vi "Unregister Event.vi"(8 "Error In":errorcluster, 9 "Registrant Address":refnum<class "Message Enqueuer.lvclass">, 10 "Event":refnum<class "Event.lvclass">, 11 "Event Source In":refnum<class "Event Source.lvclass">) -> (0 "Error Out":errorcluster, 3 "Event Source Out":refnum<class "Event Source.lvclass">)   [LabVIEW 2016, in "Event Source.lvlib" / "Event Source.lvclass"]
doc: "This method unregisters a specific Actors Enqueuer from specific Event he is listening to, in this Event Source Actor."
uses:
  Event Source.lvclass
  <vilib>/ActorFramework/Message Enqueuer/Message Enqueuer.lvclass
  Event/Event.lvclass
  Event/Event.lvclass/Event.ctl
  Event Source.lvclass/Event Source.ctl
  <resource>/AFDebug/TDM Registry.vi
  <resource>/AFDebug/Localized Strings.vi
  <resource>/AFDebug/Actor Registry.vi
  <resource>/AFDebug/Get Clone Name.vi
  <resource>/AFDebug/AF Debug.lvlib
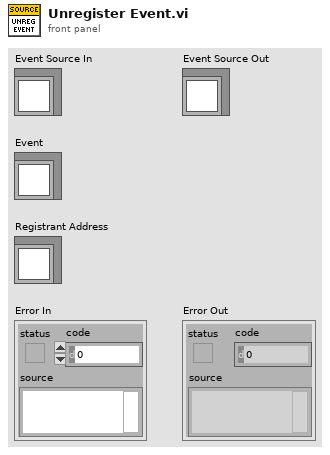
[diagram p1: front panel]
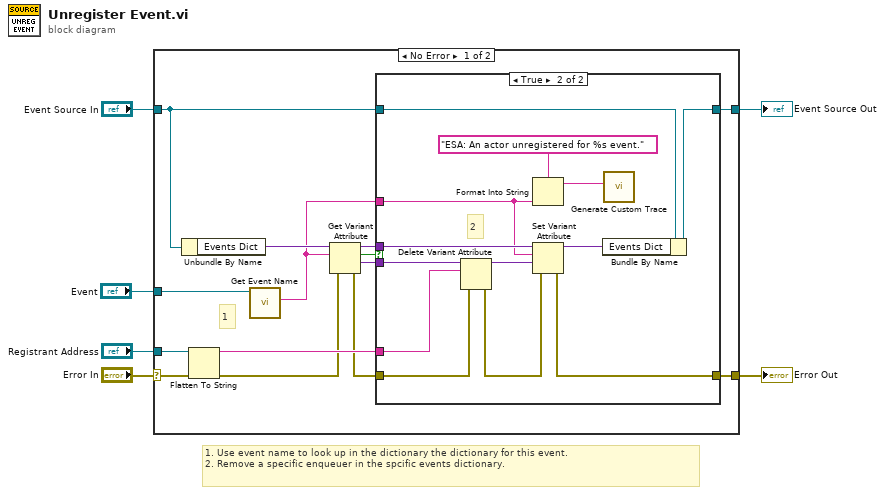
[diagram p0: block diagram]
diagram:
  # "1. Use event name to look up in the dictionary the dictionary for this event.\n2. Remove a specific enqueuer in the spcific events dictionary."
  n1 = case shown="No Error" "Error In" {
    selector: "Error In" -> [w17 w37]
    tunnel: "Registrant Address" -> [w20 _]
    tunnel: [w18 w37] -> w5
    tunnel: "Event" -> [w9 _]
    tunnel: "Event Source In" -> [w10 w36]
    tunnel: [w11 w36] -> w1
    frame No Error {
      # "1"
      n2 = Unbundle By Name(w10) -> ("Events Dict"=w16:variant)
      n3 = Flatten To String(anything=w20, error in (no error)=w17) -> (data string=w19:string, error out=w8:errorcluster)  [unwired: 2 in, 1 out]
      n4 = call "Get Event Name.vi"("Event In"=w9) -> ("Name"=w7:string)  [unwired: 9 in, 1 out]
      n5 = Get Variant Attribute(Variant=w16, name=w7, error in=w8) -> (duplicate Variant=w12:variant, found=w13:bool, value=w14:variant, error out=w15:errorcluster)  [unwired: 1 in]
      n6 = case shown="True" w13 {
        tunnel: w14 -> [_ w35]
        tunnel: w19 -> [_ w34]
        tunnel: w15 -> [w22 w33]
        tunnel: [w22 w29] -> w18
        tunnel: w12 -> [_ w32]
        tunnel: w7 -> [_ w23]
        tunnel: w10 -> [w21 w28]
        tunnel: [w21 w26] -> w11
        frame False {
        }
        frame True {
          # "2"
          n7 = Delete Variant Attribute(4:w33, 6:w34, 7:w35) -> (0:w30:errorcluster, 3:w31:variant)  [unwired: 1 out]
          n8 = Format Into String(format string="ESA: An actor unregistered for %s event." ("Custom Action"), w23) -> (resulting string=w24:string)  [unwired: 2 in, 1 out]
          n9 = Set Variant Attribute(Variant=w32, name=w23, value=w31, error in=w30) -> (Variant out=w27:variant, error out=w29:errorcluster)  [unwired: 1 out]
          n10 = Bundle By Name(cluster=w28, "Events Dict"=w27) -> (w26:refnum<class "Event Source.lvclass">)
          n11 = call <resource>:"Generate Custom Trace.vi"("Custom Action"=w24) -> ()  [unwired: 11 in]
        }
      }
    }
    frame Error {
    }
  }
  "Error Out" <- w5
  "Event Source Out" <- w1
